vi "test Loopback_Acyclic_withOverflow.vi"(8 "error in":errorcluster, 11 "TestCase in":refnum<class "Single Core Acyclic Loopback.lvclass">) -> (0 "error out":errorcluster, 3 "TestCase out":refnum<class "Single Core Acyclic Loopback.lvclass">)   [LabVIEW 2020, in "Single Core Acyclic Loopback.lvclass"]
uses:
  Single Core Acyclic Loopback.lvclass
  C:/Git/niveristand-custom-device-testing-tools/VeriStandTestCase/VeriStandTestCase.lvclass
  4b06c685-66bb-4135-9ad1-d89a50a95502.vi
  <vilib>/numeric/Random Number (Range) I64.vi
  <vilib>/numeric/sub_Random U32.vi
  <vilib>/NI VeriStand/Execution/Workspace/NI VeriStand - Set Multiple Channel Values.vi
  <vilib>/NI VeriStand/Execution/Workspace/NI VeriStand - Set Single Channel Value.vi
  <vilib>/NI VeriStand/Execution/Workspace/NI VeriStand - Get Single Channel Value.vi
  <vilib>/addons/_JKI Toolkits/VI Tester/TestCase.llb/TestCase.lvclass
  <vilib>/NI VeriStand/Execution/Workspace/NI_VS Workspace ExecutionAPI.lvlib
  C:/Program Files (x86)/National Instruments/LabVIEW 2020/vi.lib/addons/_JKI Toolkits/VI Tester/TestCase.llb/TestCase.lvclass
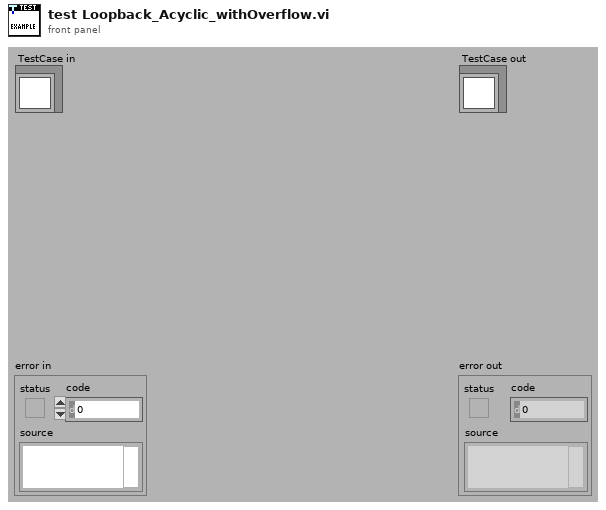
[diagram p1: front panel]
types:
  T1 = typedef "NI_VS Workspace ExecutionAPI.lvlib/WorkspaceAPI.ctl" = refnum<k24>
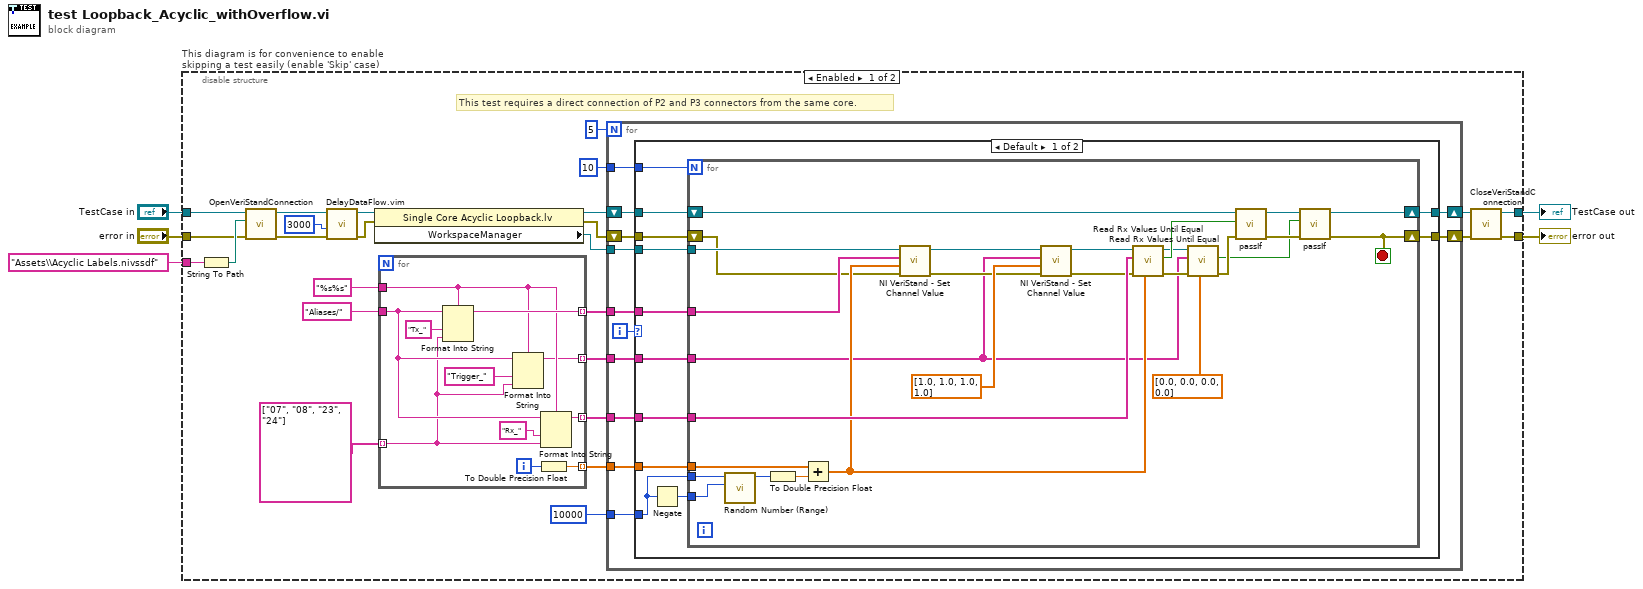
[diagram p0: block diagram]
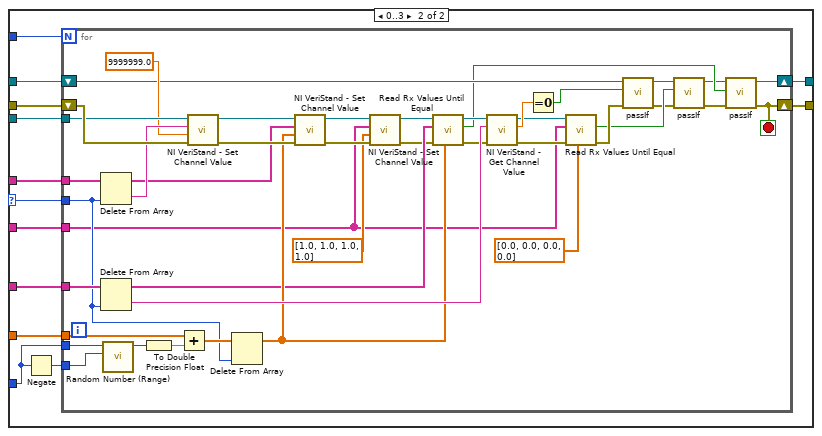
[diagram p2: hidden frame]
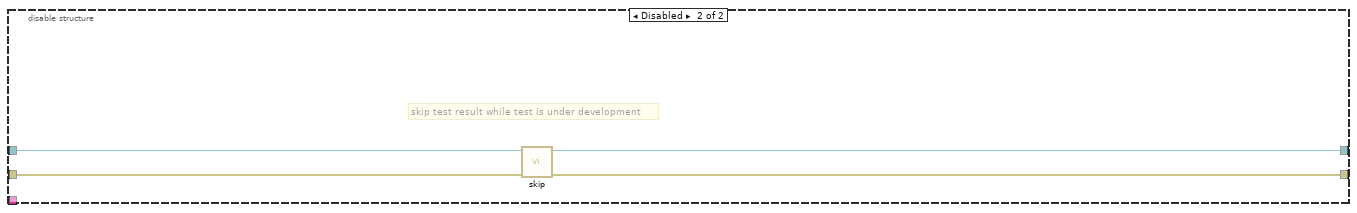
[diagram p3: hidden frame]
diagram:
  n1 = disable-structure "This diagram is for convenience to enable skipping a test easily (enable 'Skip' case)" shown="Enabled" {
    disable-tunnel: "TestCase in" -> [w25 w151]
    disable-tunnel: [w22 w149] -> w2
    disable-tunnel: [w21 w150] -> w4
    disable-tunnel: "error in" -> [w24 w148]
    disable-tunnel: "Assets\\Acyclic Labels.nivssdf" ("Channel") -> [w23 _]
    frame Enabled {
      # "This test requires a direct connection of P2 and P3 connectors from the same core."
      n2 = String To Path(string=w23) -> (path=w26:path)
      n3 = call-dynamic "OpenVeriStandConnection.vi"("error in (no error)"=w24, "System Definition File"=w26, "VeriStand Test Case in"=w25) -> ("error out"=w28:errorcluster, "VeriStand Test Case out"=w30:refnum<class "Single Core Acyclic Loopback.lvclass">)  [unwired: 6 in, 1 out]
      n4 = call "DelayDataFlow.vim"("value in"=w28, "milliseconds to wait"=u32 3000) -> ("value out"=w27:errorcluster)  [unwired: 2 in, 1 out]
      n5 = property class="Single Core Acyclic Loopback.lv"(reference=w30, error in=w27) -> (reference out=w14:refnum<class "Single Core Acyclic Loopback.lvclass">, error out=w16:errorcluster, "WorkspaceManager"=w17:T1)
      n6 = for {
        tunnel: [w147] -> w18 mode=indexing
        tunnel: [w142] -> w15 mode=indexing
        tunnel: [w146] -> w20 mode=indexing
        tunnel: "Aliases/" ("Channel") -> [w140]
        tunnel: string[] ["07", "08", "23", "24"] -> [w138] mode=indexing
        tunnel: "%s%s" ("format string") -> [w141]
        tunnel: [w137] -> w7 mode=indexing
        i -> [w145]
        n7 = Format Into String(format string=w141, initial string=w140, "Tx_" ("input 1"), w138) -> (resulting string=w147:string)  [unwired: 1 in, 1 out]
        n8 = Format Into String(format string=w141, initial string=w140, "Trigger_" ("input 1"), w138) -> (resulting string=w137:string)  [unwired: 1 in, 1 out]
        n9 = To Double Precision Float(number=w145) -> (double precision float=w146:dbl)
        n10 = Format Into String(format string=w141, initial string=w140, "Rx_" ("input 1"), w138) -> (resulting string=w142:string)  [unwired: 1 in, 1 out]
      }
      n11 = for {
        N: 5 -> [_]
        tunnel: w20 -> [w42]
        tunnel: i64 10000 ("upper bound (100)") -> [w41]
        tunnel: w18 -> [w40]
        tunnel: w17 -> [w39]
        tunnel: w15 -> [w37]
        shift-right: [w34] -> w12
        shift-left: w16 -> [w38]
        shift-right: [w35] -> w13
        shift-left: w14 -> [w36]
        tunnel: w7 -> [w32]
        tunnel: 10 -> [w31]
        i -> [w33]
        n12 = case shown="Default" w33 {
          selector: w33 -> [_ w84]
          tunnel: w42 -> [w54 w94]
          tunnel: w41 -> [w53 w93]
          tunnel: w40 -> [w51 w91]
          tunnel: w39 -> [w50 w90]
          tunnel: w38 -> [w49 w89]
          tunnel: w37 -> [w48 w88]
          tunnel: w36 -> [w47 w87]
          tunnel: [w46 w86] -> w35
          tunnel: [w45 w85] -> w34
          tunnel: w32 -> [w44 w83]
          tunnel: w31 -> [w43 w82]
          frame Default {
            n13 = Negate(x=w53) -> (-x=w52:i64)
            n14 = for {
              N: w43 -> [_]
              tunnel: w54 -> [w79]
              tunnel: w53 -> [w78]
              tunnel: w52 -> [w77]
              tunnel: w51 -> [w76]
              tunnel: w50 -> [w70]
              tunnel: w48 -> [w75]
              shift-right: [w61] -> w46
              shift-left: w47 -> [w74]
              shift-right: [w62] -> w45
              shift-left: w49 -> [w65]
              tunnel: w44 -> [w56]
              stop <- w62 stop-if-true
              n15 = call-poly <vilib>:"Random Number (Range).vi"("lower bound (-100)"=w77, "upper bound (100)"=w78) -> ("number"=w81:i64)  [unwired: 9 in]
              n16 = To Double Precision Float(number=w81) -> (double precision float=w80:dbl)
              n17 = Add(x=w79, y=w80) -> (x+y=w73:dbl[])
              n18 = call-poly <vilib>:"NI VeriStand - Set Channel Value.vi"("error in (no error)"=w65, "Values"=w73, "Channels"=w76, "WorkspaceManager in"=w70) -> ("error out"=w66:errorcluster, "WorkspaceManager out"=w69:T1)  [unwired: 6 in]
              n19 = call-poly <vilib>:"NI VeriStand - Set Channel Value.vi"("error in (no error)"=w66, "Values"=dbl[] [1.0, 1.0, 1.0, 1.0], "Channels"=w56, "WorkspaceManager in"=w69) -> ("error out"=w67:errorcluster, "WorkspaceManager out"=w68:T1)  [unwired: 6 in]
              n20 = call "Read Rx Values Until Equal.vi"("expected values"=w73, "error in"=w67, "Rx aliases"=w75, "workspace manager in"=w68) -> ("error out"=w60:errorcluster, "values equal expected"=w72:bool, "workspace manager out"=w59:T1)  [unwired: 5 in]
              n21 = call "Read Rx Values Until Equal.vi"("expected values"=dbl[] [0.0, 0.0, 0.0, 0.0] ("Values"), "error in"=w60, "Rx aliases"=w56, "workspace manager in"=w59) -> ("error out"=w58:errorcluster, "values equal expected"=w57:bool)  [unwired: 5 in, 1 out]
              n22 = call-dynamic "passIf.vi"("error in (no error)"=w58, "pass"=w72, "TestCase in"=w74) -> ("error out"=w63:errorcluster, "TestCase out"=w64:refnum<class "Single Core Acyclic Loopback.lvclass">)  [unwired: 7 in]
              n23 = call-dynamic "passIf.vi"("error in (no error)"=w63, "pass"=w57, "TestCase in"=w64) -> ("error out"=w62:errorcluster, "TestCase out"=w61:refnum<class "Single Core Acyclic Loopback.lvclass">)  [unwired: 7 in]
            }
          }
          frame 0..3 {
            n24 = Negate(x=w93) -> (-x=w92:i64)
            n25 = for {
              N: w82 -> [_]
              tunnel: w94 -> [w134]
              tunnel: w93 -> [w133]
              tunnel: w92 -> [w132]
              tunnel: w91 -> [w129]
              tunnel: w90 -> [w126]
              tunnel: w88 -> [w128]
              shift-right: [w131] -> w86
              shift-left: w87 -> [w121]
              shift-right: [w130] -> w85
              shift-left: w89 -> [w127]
              tunnel: w84 -> [w118]
              tunnel: w83 -> [w101]
              stop <- w130 stop-if-true
              n26 = Delete From Array(array=w129, index=w118) -> (deleted portion=w125:string, array with subset deleted=w113:string[])  [unwired: 1 in]
              n27 = Delete From Array(array=w128, index=w118) -> (deleted portion=w123:string, array with subset deleted=w110:string[])  [unwired: 1 in]
              n28 = call-poly <vilib>:"Random Number (Range).vi"("lower bound (-100)"=w132, "upper bound (100)"=w133) -> ("number"=w136:i64)  [unwired: 9 in]
              n29 = To Double Precision Float(number=w136) -> (double precision float=w135:dbl)
              n30 = Add(x=w134, y=w135) -> (x+y=w119:dbl[])
              n31 = call-poly <vilib>:"NI VeriStand - Set Channel Value.vi"("error in (no error)"=w127, "Value"=9999999.0, "Channel"=w125, "WorkspaceManager in"=w126) -> ("error out"=w114:errorcluster, "WorkspaceManager out"=w115:T1)  [unwired: 6 in]
              n32 = Delete From Array(array=w119, index=w118) -> (array with subset deleted=w111:dbl[])  [unwired: 1 in, 1 out]
              n33 = call-poly <vilib>:"NI VeriStand - Set Channel Value.vi"("error in (no error)"=w114, "Values"=w111, "Channels"=w113, "WorkspaceManager in"=w115) -> ("error out"=w116:errorcluster, "WorkspaceManager out"=w117:T1)  [unwired: 6 in]
              n34 = call-poly <vilib>:"NI VeriStand - Set Channel Value.vi"("error in (no error)"=w116, "Values"=dbl[] [1.0, 1.0, 1.0, 1.0], "Channels"=w101, "WorkspaceManager in"=w117) -> ("error out"=w108:errorcluster, "WorkspaceManager out"=w109:T1)  [unwired: 6 in]
              n35 = call "Read Rx Values Until Equal.vi"("expected values"=w111, "error in"=w108, "Rx aliases"=w110, "workspace manager in"=w109) -> ("error out"=w106:errorcluster, "values equal expected"=w105:bool, "workspace manager out"=w107:T1)  [unwired: 5 in]
              n36 = call-poly <vilib>:"NI VeriStand - Get Channel Value.vi"("error in (no error)"=w106, "Channel"=w123, "WorkspaceManager in"=w107) -> ("error out"=w104:errorcluster, "Value"=w122:dbl, "WorkspaceManager out"=w102:T1)  [unwired: 6 in]
              n37 = Equal To 0?(x=w122) -> (x = 0?=w120:bool)
              n38 = call "Read Rx Values Until Equal.vi"("expected values"=dbl[] [0.0, 0.0, 0.0, 0.0] ("Values"), "error in"=w104, "Rx aliases"=w101, "workspace manager in"=w102) -> ("error out"=w103:errorcluster, "values equal expected"=w99:bool)  [unwired: 5 in, 1 out]
              n39 = call-dynamic "passIf.vi"("error in (no error)"=w103, "pass"=w120, "TestCase in"=w121) -> ("error out"=w97:errorcluster, "TestCase out"=w98:refnum<class "Single Core Acyclic Loopback.lvclass">)  [unwired: 7 in]
              n40 = call-dynamic "passIf.vi"("error in (no error)"=w97, "pass"=w99, "TestCase in"=w98) -> ("error out"=w95:errorcluster, "TestCase out"=w96:refnum<class "Single Core Acyclic Loopback.lvclass">)  [unwired: 7 in]
              n41 = call-dynamic "passIf.vi"("error in (no error)"=w95, "pass"=w105, "TestCase in"=w96) -> ("error out"=w130:errorcluster, "TestCase out"=w131:refnum<class "Single Core Acyclic Loopback.lvclass">)  [unwired: 7 in]
            }
          }
        }
      }
      n42 = call-dynamic "CloseVeriStandConnection.vi"("error in (no error)"=w12, "VeriStand Test Case in"=w13) -> ("error out"=w21:errorcluster, "VeriStand Test Case out"=w22:refnum<class "Single Core Acyclic Loopback.lvclass">)  [unwired: 8 in]
    }
    frame Disabled {
      # "skip test result while test is under development"
      n43 = call <vilib>:"skip.vi"("error in (no error)"=w148, "TestCase in"=w151) -> ("error out"=w150:errorcluster, "TestCase out"=w149:refnum<class "Single Core Acyclic Loopback.lvclass">)  [unwired: 8 in]
    }
  }
  "error out" <- w4
  "TestCase out" <- w2
